vi "pc_symbol.vi"(1 "symbols":string[](array[string]), 2 "addresses":cluster{string, i64}[](array[cluster]), 3 "instruction string":string) -> (0 "address":i64)   [LabVIEW 2009]
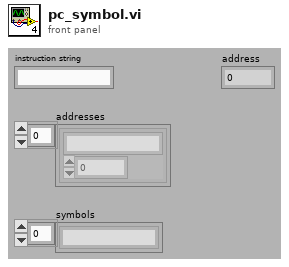
[diagram p1: front panel]
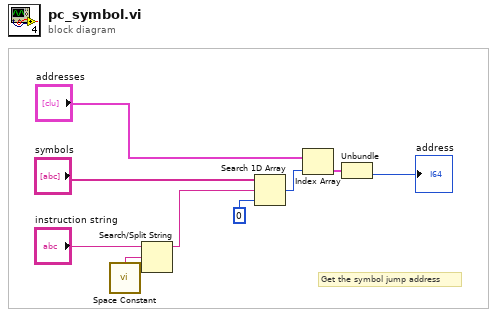
[diagram p0: block diagram]
diagram:
  # "Get the symbol jump address"
  n1 = call <vilib>:"Space Constant.vi"() -> ("String"=w2:string)
  n2 = Search/Split String(string="instruction string", search string/char (-)=w2) -> (substring before match=w1:string)  [unwired: 1 in, 2 out]
  n3 = Search 1D Array(1D array="symbols", element=w1, start index (0)=0 ("Startindex (0)")) -> (index of element=w4:i32)
  n4 = Index Array(array="addresses", index=w4) -> (element=w8:cluster{string, i64})
  n5 = Unbundle(w8) -> (→"address":i64)  [unwired: 1 out]
